vi "update.duration.request.vi"(8 "error in":errorcluster, 10 "Duration (s)":dbl, 11 "event":refnum<class "event.lvclass">) -> (0 "error out":errorcluster, 3 "request":string)   [LabVIEW 2020, in "event.lvclass"]
uses:
  event.lvclass
  event.lvclass/event.ctl
  Nominal Client/Nominal Client.lvclass
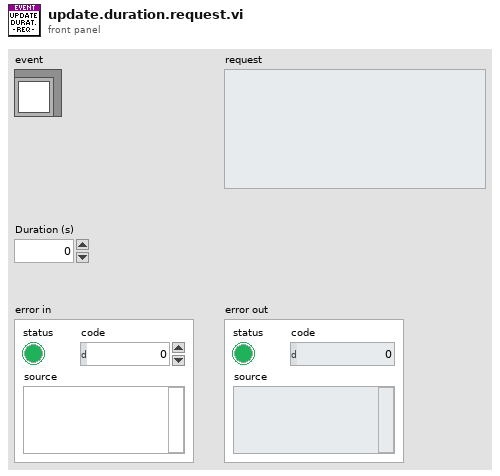
[diagram p1: front panel]
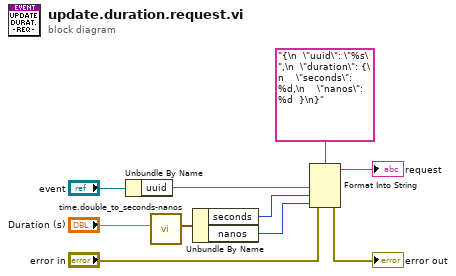
[diagram p0: block diagram]
diagram:
  n1 = Unbundle By Name("event") -> ("uuid"=w8:string)
  n2 = call "time.double_to_seconds-nanos.vi"("Time (s)"="Duration (s)") -> ("Seconds Nanos"=w2:cluster{"seconds":i32, "nanos":i32})  [unwired: 10 in]
  n3 = Unbundle By Name(w2) -> ("seconds"=w4:i32, "nanos"=w3:i32)
  n4 = Format Into String(format string="{\n  \"uuid\": \"%s\",\n  \"duration\": {\n    \"seconds\": %d,\n    \"nanos\": %d  }\n}", error in="error in", w8, w4, w3) -> (resulting string=→"request":string, error out=→"error out":errorcluster)  [unwired: 1 in]
